vi "simple_measurement.vi"() -> ()   [LabVIEW 2013]
panel:
  in  "stop":bool
  out "data 4":dbl[](array[numeric])
  out "data 3":dbl[](array[numeric])
  out "data 2":dbl[](array[numeric])
  out "element":string
  out "data":variant
  in  "OphirLMMeasurementLib.ICoLMMeasurement":refnum<k7>
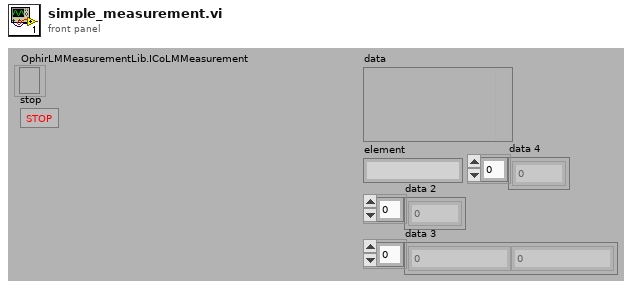
[diagram p1: front panel]
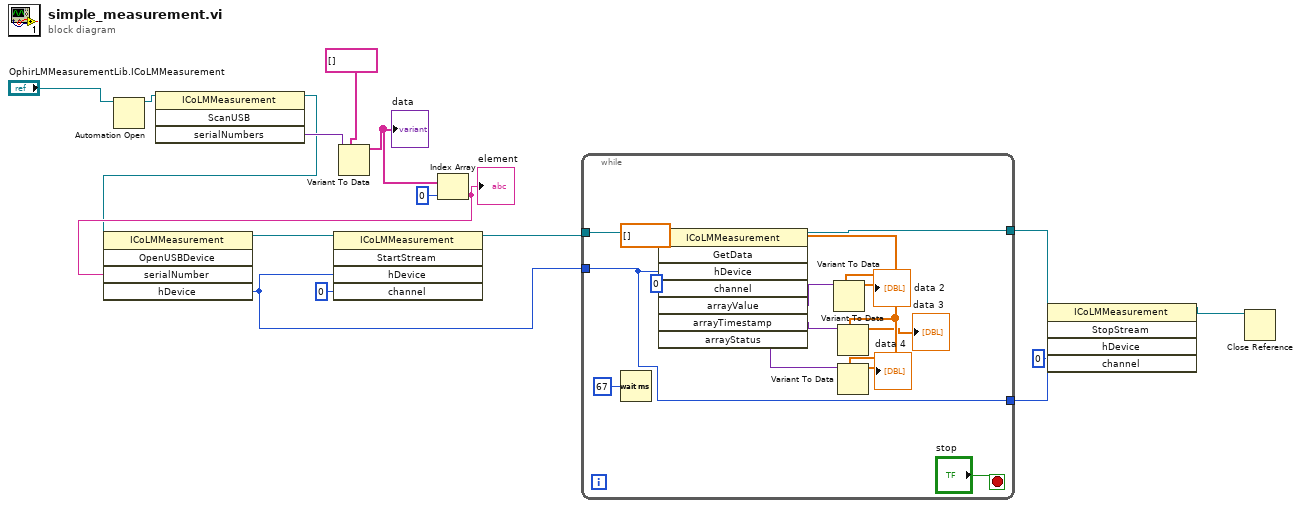
[diagram p0: block diagram]
diagram:
  n1 = Automation Open(Automation Refnum="OphirLMMeasurementLib.ICoLMMeasurement") -> (Automation Refnum=w15:refnum<k7>)  [unwired: 3 in, 1 out]
  n2 = invoke class="ICoLMMeasurement" method="ScanUSB"(reference=w15) -> (reference out=w9:refnum<k7>, "serialNumbers"=w14:variant)  [unwired: 3 in, 2 out]
  n3 = Variant To Data(type=string[] [], Variant=w14) -> (data=w13:string[])  [unwired: 1 in, 1 out]
  "data" <- w13
  n4 = Index Array(array=w13, index=0) -> (element=w10:string)
  "element" <- w10
  n5 = invoke class="ICoLMMeasurement" method="OpenUSBDevice"(reference=w9, "serialNumber"=w10) -> (reference out=w8:refnum<k7>, "hDevice"=w6:i32)  [unwired: 3 in, 3 out]
  n6 = invoke class="ICoLMMeasurement" method="StartStream"(reference=w8, "hDevice"=w6, "channel"=0) -> (reference out=w7:refnum<k7>)  [unwired: 2 in, 4 out]
  n7 = while {
    tunnel: w7 -> [w21]
    tunnel: w6 -> [w17]
    tunnel: [w18] -> w4
    tunnel: [w17] -> w3
    stop <- "stop" stop-if-true
    w25 = dbl[] []
    n8 = Wait (ms)(milliseconds to wait=u32 67) -> ()  [unwired: 1 out]
    n9 = invoke class="ICoLMMeasurement" method="GetData"(reference=w21, "hDevice"=w17, "channel"=0) -> (reference out=w18:refnum<k7>, "arrayValue"=w28:variant, "arrayTimestamp"=w27:variant, "arrayStatus"=w26:variant)  [unwired: 5 in, 4 out]
    n10 = Variant To Data(type=w25, Variant=w28) -> (data=→"data 2":dbl[])  [unwired: 1 in, 1 out]
    n11 = Variant To Data(type=w25, Variant=w27) -> (data=→"data 3":dbl[])  [unwired: 1 in, 1 out]
    n12 = Variant To Data(type=w25, Variant=w26) -> (data=→"data 4":dbl[])  [unwired: 1 in, 1 out]
  }
  n13 = invoke class="ICoLMMeasurement" method="StopStream"(reference=w4, "hDevice"=w3, "channel"=0) -> (reference out=w1:refnum<k7>)  [unwired: 2 in, 4 out]
  n14 = Close Reference(reference=w1) -> ()  [unwired: 1 in, 1 out]
